vi "求弧对应的角度.vi"(1 "r":dbl format="%#_13g", 2 "y2":dbl format="%#_13g", 3 "x2":dbl format="%#_13g", 4 "y1":dbl format="%#_13g", 5 "x1":dbl format="%#_13g") -> (0 "角度":dbl)   [LabVIEW 2016]
doc: "输入弧的起点和终点及半径 返回弧对应的角度——SEU LabVIEW CLUB"
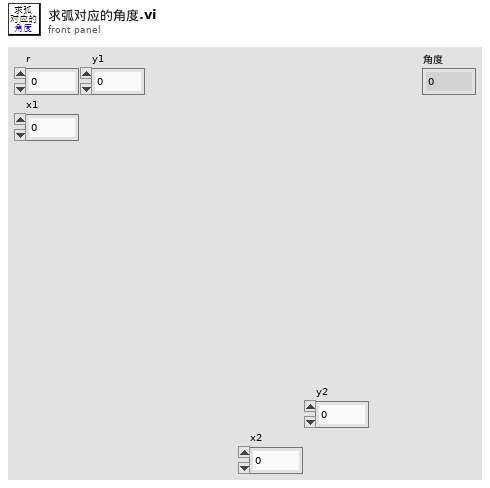
[diagram p1: front panel]
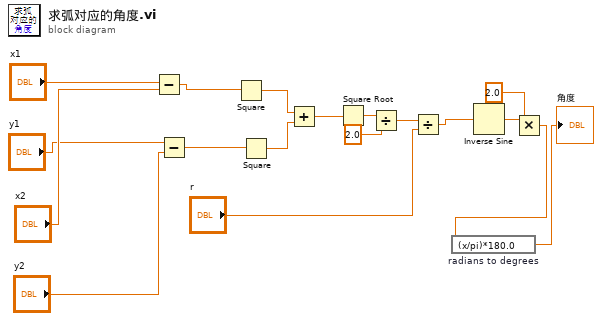
[diagram p0: block diagram]
diagram:
  n1 = Subtract(x="x1", y="x2") -> (x-y=w16:dbl)
  n2 = Subtract(x="y1", y="y2") -> (x-y=w13:dbl)
  n3 = Square(x=w16) -> (x^2=w12:dbl)
  n4 = Square(x=w13) -> (x^2=w11:dbl)
  n5 = Add(x=w12, y=w11) -> (x+y=w10:dbl)
  n6 = Square Root(x=w10) -> (sqrt(x)=w9:dbl)
  n7 = Divide(x=w9, y=2.0) -> (x/y=w7:dbl)
  n8 = Divide(x=w7, y="r") -> (x/y=w5:dbl)
  n9 = Inverse Sine(1:w5) -> (0:w4:dbl)
  n10 = Multiply(x=w4, y=2.0) -> (x*y=w2:dbl)
  n11 = expression code="(x/pi)*180.0" "radians to degrees"(w2) -> (→"角度":dbl)
